vi "Dcon Decade.vi"() -> ()   [LabVIEW 2021]
panel:
  in  "Stop Button":bool
  out "Original":cluster{dbl[], dbl[]}[](graph)
  out "XY Graph":cluster{dbl[], dbl[]}[](graph)
  in  "R*":dbl(slide) scale=-100.0..100.0
  in  "Files":path[](array[path])=[path "C:/Data/080322/m019_080322.tdms", path "C:/Data/080322/m020_080322.tdms", path "C:/Data/080322/m021_080322.tdms", path "C:/Data/080322/m022_080322.tdms", path "C:/Data/080322/m023_080322.tdms"]
  in  "Decade resistor values":dbl[](array[numeric])=[0.0, 50.0, 100.0, 150.0, 200.0]
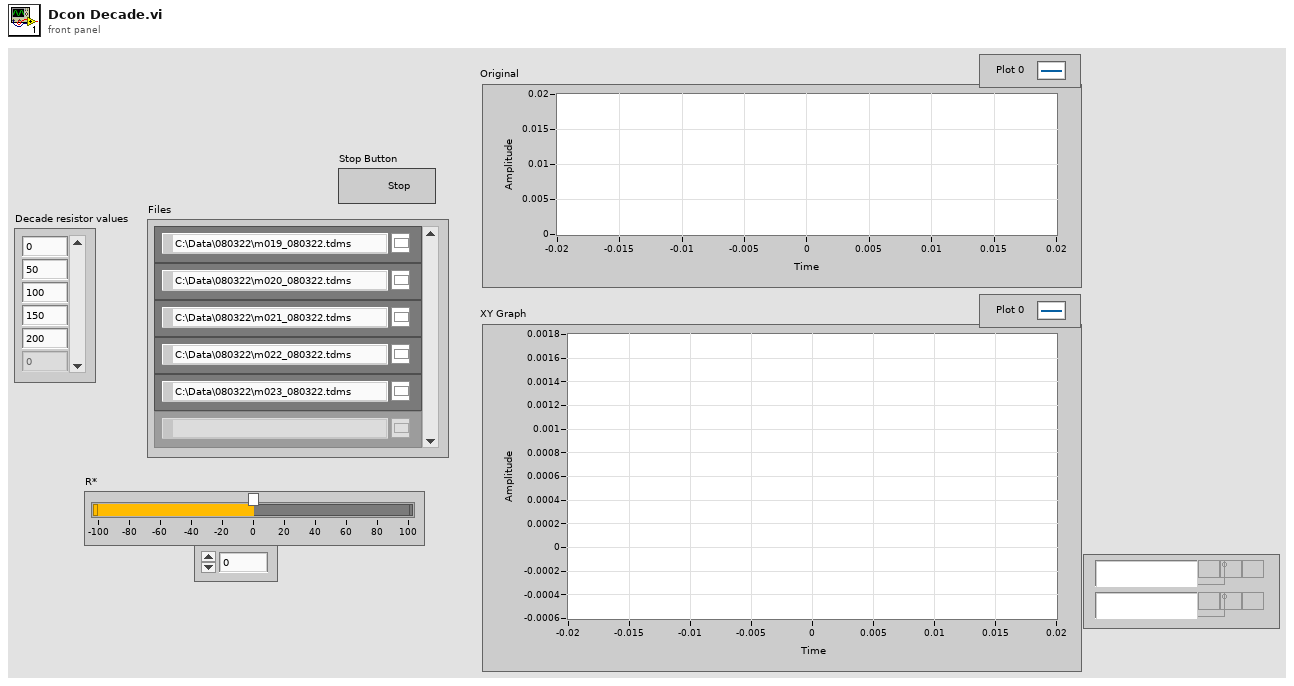
[diagram p1: front panel]
types:
  T1 = enum16{"open", "open or create", "create or replace", "create", "open (read-only)"}
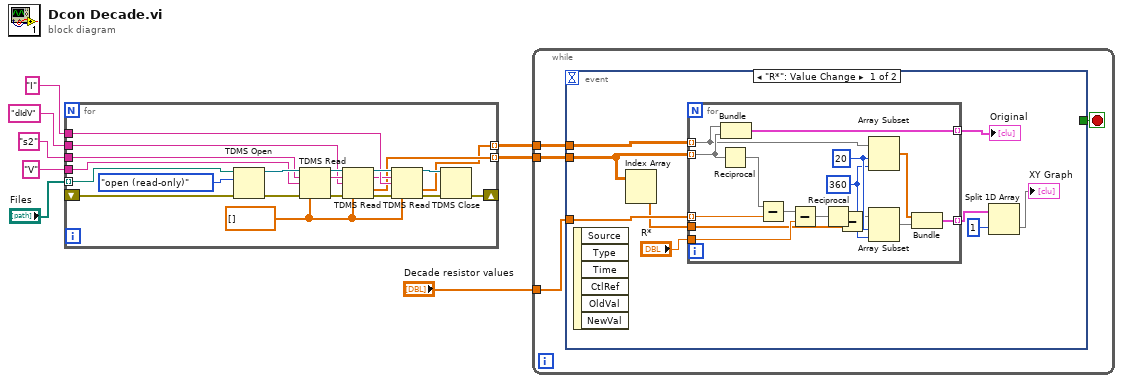
[diagram p0: block diagram]
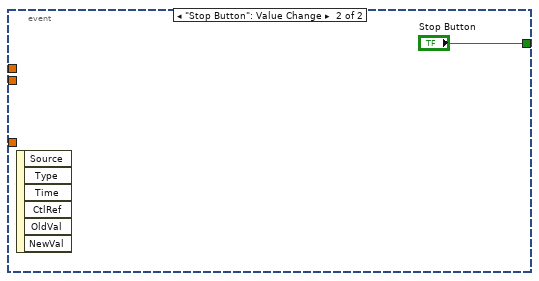
[diagram p2: hidden frame]
diagram:
  n1 = for {
    tunnel: "Files" -> [w28] mode=indexing
    shift-right: [w18] -> _
    shift-left: _ -> [w27]
    tunnel: "V" -> [w24]
    tunnel: "s2" -> [w23]
    tunnel: "dIdV" -> [w19]
    tunnel: "I" -> [w13]
    tunnel: [w10] -> w2 mode=indexing
    tunnel: [w9] -> w1 mode=indexing
    w11 = dbl[] []
    n2 = TDMS Open(8:w27, 10:T1."open (read-only)" ("operation (0:open)"), 11:w28) -> (0:w25:errorcluster, 3:w26:refnum<k34>)  [unwired: 4 in]
    n3 = TDMS Read(0:w26, 5:w23, 7:w24, 11:w25, 12:w11) -> (4:w22:refnum<k34>, 6:w21:string, 15:w20:errorcluster)  [unwired: 3 in, 3 out]
    n4 = TDMS Read(0:w22, 5:w21, 7:w19, 11:w20, 12:w11) -> (4:w15:refnum<k34>, 6:w12:string, 10:w10:dbl[], 15:w17:errorcluster)  [unwired: 3 in, 2 out]
    n5 = TDMS Read(0:w15, 5:w12, 7:w13, 11:w17, 12:w11) -> (4:w14:refnum<k34>, 10:w9:dbl[], 15:w16:errorcluster)  [unwired: 3 in, 3 out]
    n6 = TDMS Close(8:w16, 11:w14) -> (0:w18:errorcluster)  [unwired: 1 out]
  }
  n7 = while {
    tunnel: "Decade resistor values" -> [w33]
    tunnel: w2 -> [w32]
    tunnel: w1 -> [w31]
    stop <- w30 stop-if-true
    n8 = event shown="[0] \"R*\": Value Change" {
      selector: _ -> [_ _]
      dyn-events: _ -> [_ _]
      timeout: _ -> [_ _]
      tunnel: w33 -> [w42 _]
      tunnel: w32 -> [w38 _]
      tunnel: w31 -> [w41 _]
      tunnel: [_ "Stop Button"] -> w30
      event "R*": Value Change {
        n9 = event-data() -> ()  [unwired: 1 in, 6 out]
        n10 = Index Array(array=w38) -> (element=w37:dbl[])  [unwired: 2 in]
        n11 = for {
          tunnel: w42 -> [w57] mode=indexing
          tunnel: w38 -> [w52] mode=indexing
          tunnel: "R*" -> [w55]
          tunnel: w41 -> [w50] mode=indexing
          tunnel: [w53] -> w35 mode=indexing
          tunnel: [w51] -> w40 mode=indexing
          tunnel: w37 -> [w43]
          w47 = 360 ("length")
          w48 = 20 ("length")
          n12 = Reciprocal(x=w52) -> (1/x=w58:dbl[])
          n13 = Bundle(w50, w52) -> (w51:cluster{dbl[], dbl[]})  [unwired: 1 in]
          n14 = Subtract(x=w58, y=w57) -> (x-y=w56:dbl[])
          n15 = Subtract(x=w56, y=w55) -> (x-y=w54:dbl[])
          n16 = Reciprocal(x=w54) -> (1/x=w46:dbl[])
          n17 = Subtract(x=w46, y=w43) -> (x-y=w44:dbl[])
          n18 = Array Subset(array=w50, index=w48, length=w47) -> (w49:dbl[])
          n19 = Array Subset(array=w44, index=w48, length=w47) -> (w45:dbl[])
          n20 = Bundle(w49, w45) -> (w53:cluster{dbl[], dbl[]})  [unwired: 1 in]
        }
        "Original" <- w40
        n21 = Split 1D Array(array=w35, index=1) -> (second subarray=→"XY Graph":cluster{dbl[], dbl[]}[])  [unwired: 1 out]
      }
      event "Stop Button": Value Change {
        n22 = event-data() -> ()  [unwired: 1 in, 6 out]
      }
    }
  }
